vi "Write Unique Identifier.vi"(8 "error in (no error)":errorcluster, 10 "Unique Identifier":string, 11 "Measurement Done in":refnum<class "Measurement Done.lvclass">) -> (0 "error out":errorcluster, 3 "Measurement Done out":refnum<class "Measurement Done.lvclass">)   [LabVIEW 2017, in "Controller Actor.lvlib" / "Measurement Done.lvclass"]
uses:
  Measurement Done.lvclass
  Measurement Done.lvclass/Measurement Done.ctl
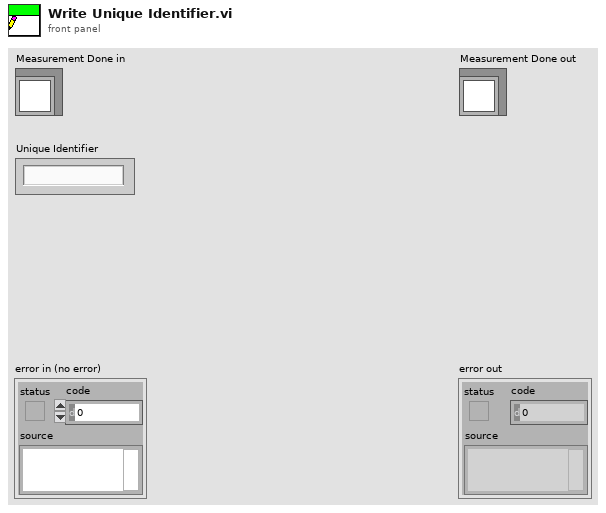
[diagram p1: front panel]
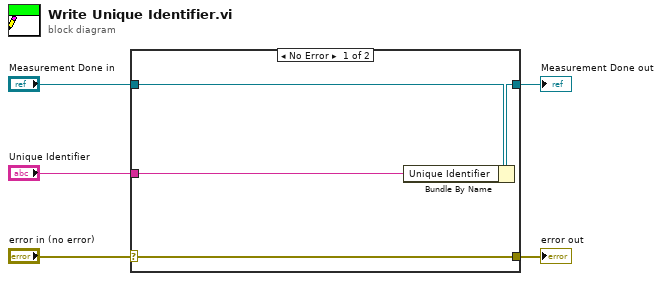
[diagram p0: block diagram]
diagram:
  n1 = case shown="No Error" "error in (no error)" {
    selector: "error in (no error)" -> [w9 w10]
    tunnel: [w9 w10] -> w4
    tunnel: [w7 w11] -> w2
    tunnel: "Measurement Done in" -> [w8 w11]
    tunnel: "Unique Identifier" -> [w6 _]
    frame No Error {
      n2 = Bundle By Name(cluster=w8, "Unique Identifier"=w6) -> (w7:refnum<class "Measurement Done.lvclass">)
    }
    frame Error {
    }
  }
  "error out" <- w4
  "Measurement Done out" <- w2
